vi "Main FPGA 5-axis with 5AxisLimitU8 48DIO.vi"() -> ()   [LabVIEW 2013]
uses:
  <vilib>/Motion/MotorControl/_s/nism.interpretControlRegister.stateTransition.ctl
  <vilib>/Platform/TimedLoop/XDataNode/timing_clust.ctl
  <vilib>/Platform/TimedLoop/XDataNode/nitl_modes.ctl
  <vilib>/Platform/TimedLoop/XDataNode/wakeup.ctl
  <vilib>/Motion/MotorControl/_s/nism.digitalInputs.portA.ctl
  <vilib>/rvi/Emulation/niFpgaSctlEmulationGetInTimedLoop.vi
  <vilib>/rvi/Emulation/niFpgaEmulationReportErrorSimple.vi
  <vilib>/rvi/Emulation/niFpgaGetClockAttributes.vi
  <vilib>/rvi/Emulation/niFpgaCriticalErrorInLSC.vi
  Global FPGA.vi
  <vilib>/rvi/eio/common/nirviEmuTemplateMethod_errors.vi
  <vilib>/Motion/SoftMotion/Synchronization/nism.rioScan.generateSyncScan.vi
  <vilib>/rvi/Emulation/niFpgaProcessEmulError.vi
  <vilib>/Motion/MotorControl/_s/nism.interpretControlRegister.indexed.vi
  <vilib>/Motion/MotorControl/_s/nism.generateStatusRegister.indexed.vi
  <vilib>/Motion/MotorControl/_s/nism.mdo.read.positionLoopSyncData.vi
  <vilib>/Motion/MotorControl/_s/nism.mdo.read.splineData.vi
  <vilib>/Motion/MotorControl/_s/nism.splineInterpolation.fxp.3.index.vi
  <vilib>/Motion/MotorControl/_s/nism.mdo.handler.indexed.vi
  <vilib>/Motion/MotorControl/_s/nism.interpretDIOControl.portA.single.2.vi
  <vilib>/Motion/MotorControl/_s/nism.generateDIOStatus.portA.single.vi
  <vilib>/Platform/TimedLoop/XDataNode/XDataNode.xnode
  <vilib>/eio/EIONode/EIONode.xnode
  <vilib>/Motion/MotorControl/NI_SoftMotion_MotorControlIP.lvlib
  <vilib>/Platform/TimedLoop/XDataNode/XDNodeRunTimeDep.lvlib
  <vilib>/Motion/SoftMotion/Synchronization/NI_SoftMotion_Synchronization.lvlib
panel:
  out "DI (24bits)":u32
  in  "DO (24bits)":u32
  in  "Axis Digital Input":u8[](array[numeric])=[0, 0, 0, 0, 0]
  out "Axis Positions":fxp<+/-,64,32>[](array[numeric])
  in  "STEP or CW? (T=STEP)":bool
  out "Drive Enable":bool[](array[boolean])
  in  "Enable Watchdog":bool
  in  "Pet Watchdog":bool
  in  "Watchdog Timeout Period (ticks)":u64=40000000 format="%.0p"
  out "Watchdog Timed Out?":bool
  out "Time Since Last Pet":u64
  in  "Enable value":bool
  in  "Drive Enable override?":bool
  out "State":T1=enum."Start --> Initializing" caption="state transition"
  in  "Sync Value":bool
  in  "Sync Enable override?":bool
  in  "Invert direction?":bool
  out "Sync is Fault":bool
  out "Sync is Locked":bool
  in  "minimum pulse":u16=40
  # "Synchronization Loop"
  # "Control Status Loop"
  # "Notes: \n1. This VI provides the communication interface between the NI SoftMotion Engine and the LabVIEW FPGA Module. You must compile this VI for a specific FPGA target before use. After compiling, run the VI before running any of the Express VI examples. For information on moving this example to another FPGA target, refer to ni.com/info and enter info code fpgaex.\n\n2. Only use the Reset Axis button if you are unable to communicate with the axis by any other means. This button resets the device state machine and other VIs to a known state. After resetting the axis, switch the NI Scan Engine from Active Mode to Configuration Mode, then back to Active Mode, before attempting to enable the axis."
  # "(These two buttons \nare for testing\npurposes.)"
  # "(These two buttons \nare for testing\npurposes.)"
  # "Step/Direction Loop"
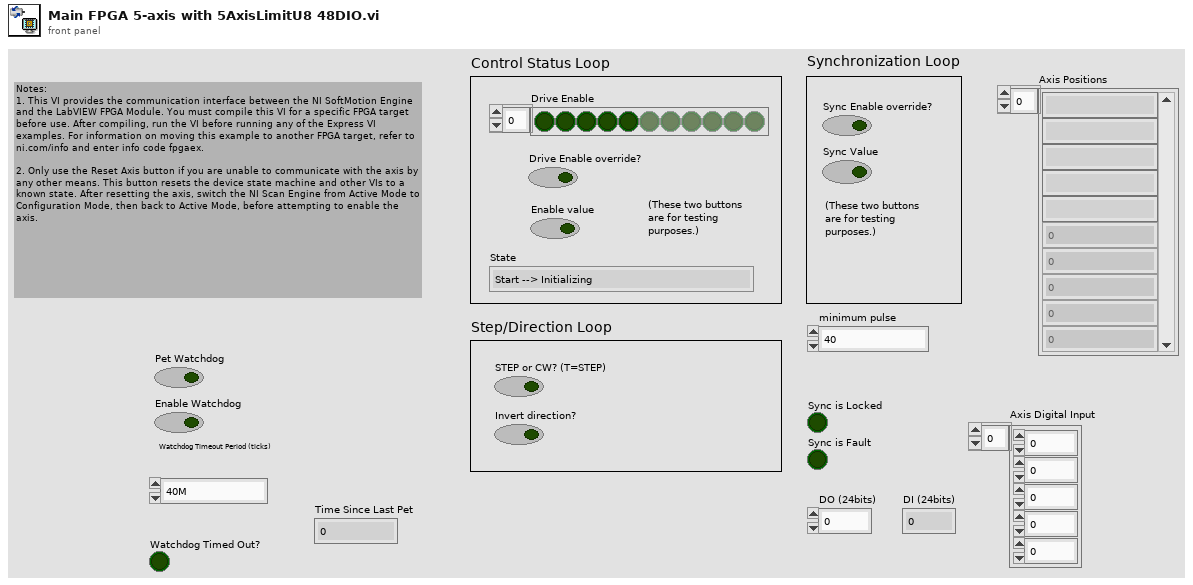
[diagram p1: front panel]
types:
  T1 = typedef "NI_SoftMotion_MotorControlIP.lvlib/nism.interpretControlRegister.stateTransition.ctl" = enum8{"Invalid", "Start --> Initializing", "Initializing --> Disabled", "Disabled --> Ready To Switch On", "Ready To Switch On --> Switched On", "Ready To Switch On --> Disable", "Switched On --> Operation Enable", "Switched On --> Ready To Switch On", "Switched On --> Disabled", "Operation Enable --> Switched On", "Operation Enable --> Ready To Switch On", "Operation Enable --> Disabled", "Fault --> Disabled", "Any --> Fault", "None"}
  T2 = typedef "NI_SoftMotion_MotorControlIP.lvlib/nism.mdo.splineData.ctl" = cluster{"spline type":T3, "traj per/spline per":u16, "spline per/traj per":fxp<+,32,0>}
  T3 = typedef "nism.splineInterpolation.type.ctl" = u16
  T4 = typedef "NI_SoftMotion_Synchronization.lvlib/nism.softmotionScan.timerConfig.ctl" = cluster{"Target Period (clocks)":u16, "Host Period / Target Period":u16}
  T5 = typedef "NI_SoftMotion_MotorControlIP.lvlib/nism.digitalInputs.portA.ctl" = cluster{"reverse limit":bool, "forward limit":bool, "home switch":bool, "digital input 0":bool, "digital input 1":bool, "digital input 2":bool, "digital input 3":bool}
  T6 = typedef "NI_SoftMotion_MotorControlIP.lvlib/nism.dio.portA.config.2.ctl" = cluster{"digital filter (us)":u16[], "safe state":enum16{"Low", "High", "No Change"}[]}
  T7 = typedef "XDNodeRunTimeDep.lvlib/timing_clust.ctl" = cluster{"Expected End [f-1]":u64, "Actual End [f-1]":u64, "Finished Late? [f-1]":bool, "Expected End [i-1]":u64, "Actual End [i-1]":u64, "Finished Late? [i-1]":bool, "Expected Start [i]":u64, "Actual Start [i]":u64, "Expected Start [f]":u64, "Actual Start [f]":u64, "Source Name":string, "Structure Name":string, "Period":i64, "Deadline":i64, "Offset":i64, "Start":i64, "Priority":i32, "Timeout":i32, "Mode":T8, "Wakeup Reason":T9, "Error":errorcluster, "Source Type":string, "Secondary Source Type":string, "Global End Time":u64, "Global Start Time":u64, "Frame Duration":u64, "Iteration Duration":u64, "Assigned CPU":i32, "I/O Scan Engine Mode":u32}
  T8 = typedef "XDNodeRunTimeDep.lvlib/nitl_modes.ctl" = enum32{"No Change", "Process missed periods, maintain original phase", "Discard missed periods, maintain original phase", "Process missed periods, ignore original phase", "Discard missed periods, ignore original phase"}
  T9 = typedef "XDNodeRunTimeDep.lvlib/wakeup.ctl" = enum32{"Normal", "Aborted", "Asynchronous wakeup", "Timing source error", "Timed loop error", "Timeout"}
  T10 = typedef "NI_SoftMotion_Synchronization.lvlib/nism.softmotionScan.timerControl.ctl" = cluster{"SM Scan":bool, "SM Scan Count":u32, "SM Scan Enabled":bool}
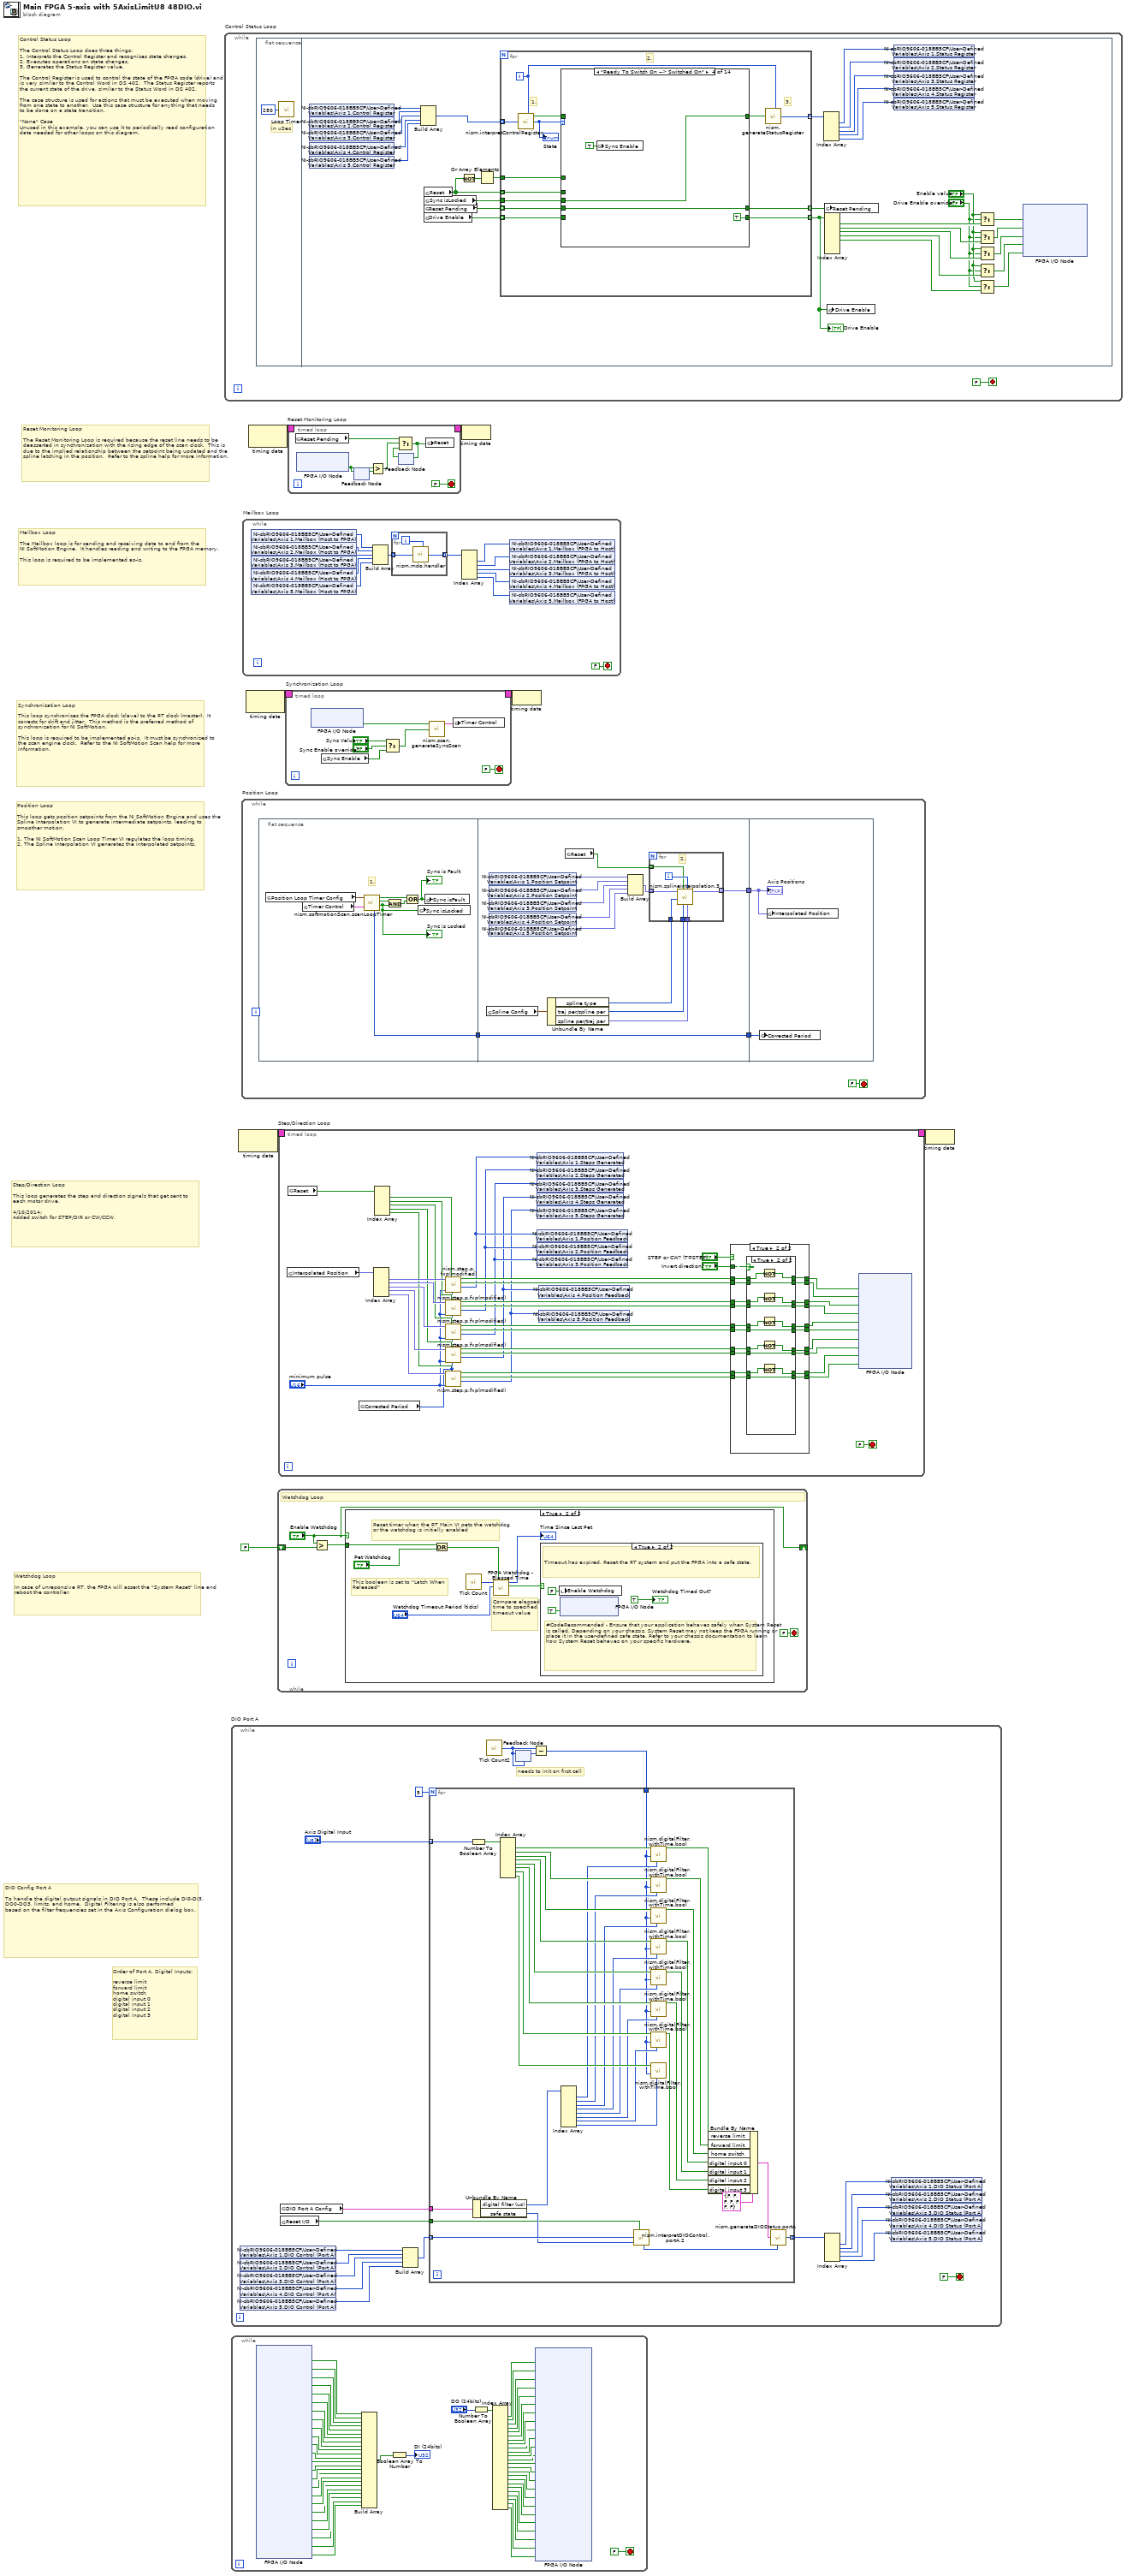
[diagram p0: block diagram]
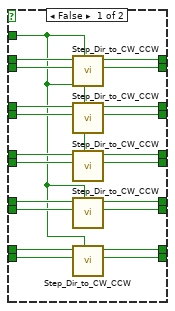
[diagram p4: hidden frame]
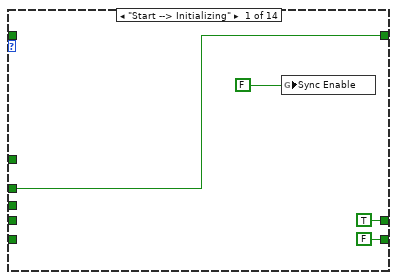
[diagram p6: hidden frame]
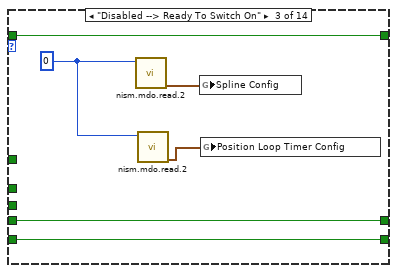
[diagram p8: hidden frame]
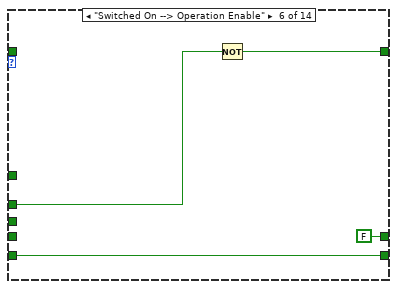
[diagram p10: hidden frame]
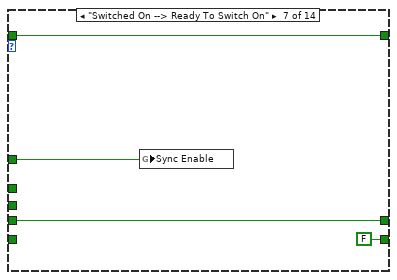
[diagram p11: hidden frame]
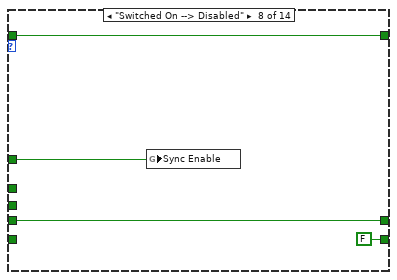
[diagram p12: hidden frame]
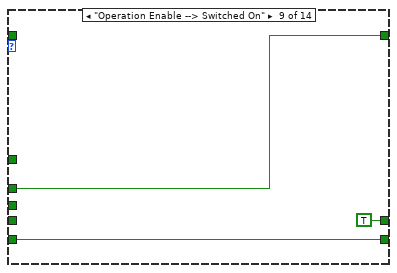
[diagram p13: hidden frame]
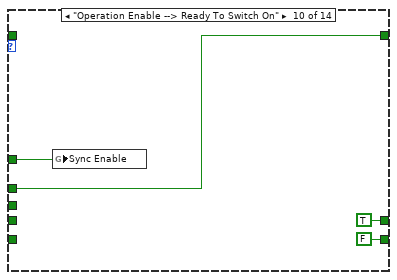
[diagram p14: hidden frame]
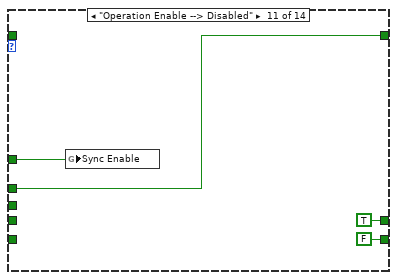
[diagram p15: hidden frame]
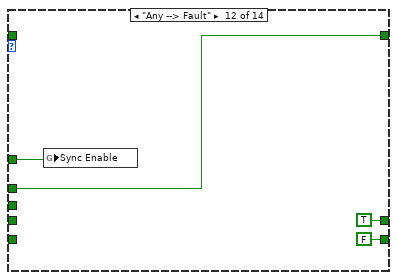
[diagram p16: hidden frame]
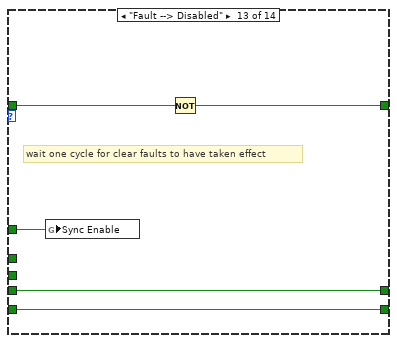
[diagram p17: hidden frame]
diagram:
  # "DIO Config Port A\n\nTo handle the digital output signals in DIO Port A.  These include DI0-DI3, DO0-DO3, limits, and home.  Digital Filtering is also performed\nbased on the filter frequencies set in the Axis Configuration dialog box."
  # "Order of Port A, Digital Inputs:\n\nreverse limit\nforward limit\nhome switch\ndigital input 0\ndigital input 1\ndigital input 2\ndigital input 3"
  # "Watchdog Loop\n\nIn case of unreponsive RT, the FPGA will assert the \"System Reset\" line and reboot the controller."
  # "Step/Direction Loop\n\nThis loop generates the step and direction signals that get sent to \neach motor drive.\n\n4/10/2014:\nAdded switch for STEP/DIR or CW/CCW."
  # "Position Loop\n\nThis loop gets position setpoints from the NI SoftMotion Engine and uses the Spline Interpolation VI to generate intermediate setpoints, leading to smoother motion.\n\n1. The NI SoftMotion Scan Loop Timer VI regulates the loop timing. \n2. The Spline Interpolation VI generates the interpolated setpoints."
  # "Synchronization Loop\n\nThis loop synchronizes the FPGA clock (slave) to the RT clock (master).  It corrects for drift and jitter.  This method is the preferred method of synchronization for NI SoftMotion.\n\nThis loop is required to be implemented as-is.  It must be synchronized to the scan engine clock.  Refer to the NI SoftMotion Scan help for more information."
  # "Mailbox Loop\n\nThe Mailbox loop is for sending and receiving data to and from the \nNI SoftMotion Engine.  It handles reading and writing to the FPGA memory.\n\nThis loop is required to be implemented as-is."
  # "Reset Monitoring Loop\n\nThe Reset Monitoring Loop is required because the reset line needs to be deasserted in synchronization with the rising edge of the scan clock.  This is due to the implied relationship between the setpoint being updated and the spline latching in the position.  Refer to the spline help for more information."
  # "Control Status Loop\n\nThe Control Status Loop does three things:\n1. Interprets the Control Register and recognizes state changes.\n2. Executes operations on state changes.\n3. Generates the Status Register value.\n\nThe Control Register is used to control the state of the FPGA code (drive) and is very similar to the Control Word in DS 402.  The Status Register reports the current state of the drive, similar to the Status Word in DS 402.\n\nThe case structure is used for actions that must be executed when moving from one state to another.  Use this case structure for anything that needs to be done on a state transition.\n\n\"None\" Case\nUnused in this example, you can use it to periodically read configuration data needed for other loops on this diagram."
  n1 = while "Control Status Loop" {
    stop <- FALSE stop-if-true
    n2 = flat-sequence {
      frame #0 {
        # "in uSec"
        n3 = call "Loop Timer"("Count(uSec)"=u32 250) -> ()  [unwired: 1 out]
      }
      frame #1 {
        n4 = shared-variable "NI-sbRIO9606-018BB5CF\\User-Defined Variables\\Axis 1.Control Register"() -> (w31:u32)  [unwired: 1 in, 1 out]
        n5 = shared-variable "NI-sbRIO9606-018BB5CF\\User-Defined Variables\\Axis 2.Control Register"() -> (w30:u32)  [unwired: 1 in, 1 out]
        n6 = shared-variable "NI-sbRIO9606-018BB5CF\\User-Defined Variables\\Axis 3.Control Register"() -> (w29:u32)  [unwired: 1 in, 1 out]
        n7 = shared-variable "NI-sbRIO9606-018BB5CF\\User-Defined Variables\\Axis 4.Control Register"() -> (w28:u32)  [unwired: 1 in, 1 out]
        n8 = shared-variable "NI-sbRIO9606-018BB5CF\\User-Defined Variables\\Axis 5.Control Register"() -> (w27:u32)  [unwired: 1 in, 1 out]
        n9 = Build Array(w31, w30, w29, w28, w27) -> (w40:u32[])
        n10 = global read "Global FPGA.vi" "Reset Pending"() -> (w35:bool[])
        n11 = global read "Global FPGA.vi" "Drive Enable"() -> (w34:bool[])
        n12 = global read "Global FPGA.vi" "Reset"() -> (w36:bool[])
        n13 = global read "Global FPGA.vi" "Sync isLocked"() -> (w41:bool)
        n14 = Not(x=w36) -> (.not. x?=w38:bool[])
        n15 = Or Array Elements(Boolean array=w38) -> (logical OR=w37:bool)
        n16 = for {
          tunnel: w36 -> [w49] mode=indexing
          tunnel: w41 -> [w48]
          tunnel: w40 -> [w50] mode=indexing
          tunnel: [w47] -> w32 mode=indexing
          tunnel: [w46] -> w39 mode=indexing
          tunnel: [w45] -> w33 mode=indexing
          tunnel: w37 -> [w44]
          tunnel: w35 -> [w43] mode=indexing
          tunnel: w34 -> [w42] mode=indexing
          i -> [w51]
          # "3."
          # "2."
          # "1."
          n17 = call-poly <vilib>:"nism.interpretControlRegister.vi"("control register"=w50, "axis index"=w51) -> ("transition occurred"=w52:bool, "state transition"=w53:T1)  [unwired: 6 in]
          "State" <- w53
          n18 = case shown="\"Ready To Switch On --> Switched On\"" w53 {
            tunnel: w52 -> [_ w61 w67 _ w74 _ w82 w86 _ _ _ _ w106 _]
            tunnel: [w58 w61 w67 w69 w74 w78 w82 w86 w88 w91 w95 w99 w105 _] -> w54
            tunnel: w49 -> [w58 _ _ _ _ w77 _ _ w88 w91 w95 w99 _ _]
            tunnel: w48 -> [_ _ _ w69 _ _ _ _ _ _ _ _ _ _]
            tunnel: [TRUE ("Write.Reset Pending") w60 w63 w68 w73 FALSE ("Write.Reset Pending") w79 w83 TRUE ("Write.Reset Pending") TRUE ("Write.Reset Pending") TRUE ("Write.Reset Pending") TRUE ("Write.Reset Pending") w103 w108] -> w46
            tunnel: [FALSE ("Write.Drive Enable") w59 w62 TRUE ("Write.Drive Enable") w72 w75 FALSE ("Write.Drive Enable") FALSE ("Write.Drive Enable") w87 FALSE ("Write.Drive Enable") FALSE ("Write.Drive Enable") FALSE ("Write.Drive Enable") w102 w107] -> w45
            tunnel: w44 -> [_ _ _ _ _ _ w80 w84 _ w90 w94 w98 w104 _]
            tunnel: w43 -> [_ w60 w63 w68 w73 _ w79 w83 _ _ _ _ w103 w108]
            tunnel: w42 -> [_ w59 w62 _ w72 w75 _ _ w87 _ _ _ w102 w107]
            frame "Start --> Initializing" {
              n19 = global write "Global FPGA.vi" "Sync Enable"(FALSE ("Sync Enable")) -> ()
            }
            frame "Initializing --> Disabled" {
            }
            frame "Disabled --> Ready To Switch On" {
              w65 = 0 ("axis index")
              n20 = call-poly <vilib>:"nism.mdo.read.2.vi"("axis index"=w65) -> ("spline"=w66:T2)  [unwired: 10 in]
              n21 = call-poly <vilib>:"nism.mdo.read.2.vi"("axis index"=w65) -> ("position loop sync"=w64:T4)  [unwired: 10 in]
              n22 = global write "Global FPGA.vi" "Spline Config"(w66) -> ()
              n23 = global write "Global FPGA.vi" "Position Loop Timer Config"(w64) -> ()
            }
            frame "Ready To Switch On --> Switched On" {
              n24 = global write "Global FPGA.vi" "Sync Enable"(TRUE ("Sync Enable")) -> ()
            }
            frame "Ready To Switch On --> Disable" {
            }
            frame "Switched On --> Operation Enable" {
              n25 = Not(x=w77) -> (.not. x?=w78:bool)
            }
            frame "Switched On --> Ready To Switch On" {
              n26 = global write "Global FPGA.vi" "Sync Enable"(w80) -> ()
            }
            frame "Switched On --> Disabled" {
              n27 = global write "Global FPGA.vi" "Sync Enable"(w84) -> ()
            }
            frame "Operation Enable --> Switched On" {
            }
            frame "Operation Enable --> Ready To Switch On" {
              n28 = global write "Global FPGA.vi" "Sync Enable"(w90) -> ()
            }
            frame "Operation Enable --> Disabled" {
              n29 = global write "Global FPGA.vi" "Sync Enable"(w94) -> ()
            }
            frame "Any --> Fault" {
              n30 = global write "Global FPGA.vi" "Sync Enable"(w98) -> ()
            }
            frame "Fault --> Disabled" {
              # "wait one cycle for clear faults to have taken effect"
              n31 = global write "Global FPGA.vi" "Sync Enable"(w104) -> ()
              n32 = Not(x=w106) -> (.not. x?=w105:bool)
            }
            frame "None", Default {
            }
          }
          n33 = call-poly <vilib>:"nism.generateStatusRegister.vi"("transition success"=w54, "axis index"=w51) -> ("status register"=w47:u32)  [unwired: 7 in]
        }
        "Drive Enable" <- w33
        n34 = Index Array(array=w32) -> (element #1=w26:u32, element #2=w25:u32, element #3=w24:u32, element #4=w23:u32, element #5=w22:u32)  [unwired: 5 in]
        n35 = global write "Global FPGA.vi" "Reset Pending"(w39) -> ()
        n36 = Index Array(array=w33) -> (element #1=w21:bool, element #2=w19:bool, element #3=w17:bool, element #4=w15:bool, element #5=w13:bool)  [unwired: 8 in, 3 out]
        n37 = global write "Global FPGA.vi" "Drive Enable"(w33) -> ()
        n38 = shared-variable "NI-sbRIO9606-018BB5CF\\User-Defined Variables\\Axis 1.Status Register"(w26) -> ()  [unwired: 1 in, 1 out]
        n39 = shared-variable "NI-sbRIO9606-018BB5CF\\User-Defined Variables\\Axis 2.Status Register"(w25) -> ()  [unwired: 1 in, 1 out]
        n40 = shared-variable "NI-sbRIO9606-018BB5CF\\User-Defined Variables\\Axis 3.Status Register"(w24) -> ()  [unwired: 1 in, 1 out]
        n41 = shared-variable "NI-sbRIO9606-018BB5CF\\User-Defined Variables\\Axis 4.Status Register"(w23) -> ()  [unwired: 1 in, 1 out]
        n42 = shared-variable "NI-sbRIO9606-018BB5CF\\User-Defined Variables\\Axis 5.Status Register"(w22) -> ()  [unwired: 1 in, 1 out]
        n43 = Select(t="Enable value", s="Drive Enable override?", f=w21) -> (s? t:f=w20:bool)
        n44 = Select(t="Enable value", s="Drive Enable override?", f=w19) -> (s? t:f=w18:bool)
        n45 = Select(t="Enable value", s="Drive Enable override?", f=w17) -> (s? t:f=w16:bool)
        n46 = Select(t="Enable value", s="Drive Enable override?", f=w15) -> (s? t:f=w14:bool)
        n47 = Select(t="Enable value", s="Drive Enable override?", f=w13) -> (s? t:f=w12:bool)
        n48 = xnode "FPGA I/O Node"("Axis1_Servo On"=w20, "Axis2_Servo On"=w18, "Axis3_Servo On"=w16, "Axis4_Servo On"=w14, "Axis5_Servo On"=w12) -> ()  [unwired: 5 in, 5 out]
      }
    }
  }
  n49 = while "DIO Port A" {
    stop <- FALSE stop-if-true
    # "needs to init on first call"
    n50 = shared-variable "NI-sbRIO9606-018BB5CF\\User-Defined Variables\\Axis 1.DIO Control (Port A)"() -> (w125:u32)  [unwired: 1 in, 1 out]
    n51 = shared-variable "NI-sbRIO9606-018BB5CF\\User-Defined Variables\\Axis 2.DIO Control (Port A)"() -> (w124:u32)  [unwired: 1 in, 1 out]
    n52 = shared-variable "NI-sbRIO9606-018BB5CF\\User-Defined Variables\\Axis 3.DIO Control (Port A)"() -> (w123:u32)  [unwired: 1 in, 1 out]
    n53 = shared-variable "NI-sbRIO9606-018BB5CF\\User-Defined Variables\\Axis 4.DIO Control (Port A)"() -> (w122:u32)  [unwired: 1 in, 1 out]
    n54 = shared-variable "NI-sbRIO9606-018BB5CF\\User-Defined Variables\\Axis 5.DIO Control (Port A)"() -> (w121:u32)  [unwired: 1 in, 1 out]
    n55 = global read "Global FPGA.vi" "DIO Port A Config"() -> (w109:T6)
    n56 = global read "Global FPGA.vi" "Reset I/O"() -> (w110:bool)
    n57 = Build Array(w125, w124, w123, w122, w121) -> (w120:u32[])
    n58 = call "Tick Count2"() -> ("Tick Count(uSec)"=w113:u16)
    n59 = feedback #1(w113) -> (w112:u16)
    n60 = feedback-in #1(w113) -> ()
    n61 = Subtract(x=w113, y=w112) -> (x-y=w111:u16)
    n62 = for {
      N: 5 -> [_]
      tunnel: [w162] -> w114 mode=indexing
      tunnel: w120 -> [w161] mode=indexing
      tunnel: w109 -> [w158]
      tunnel: w110 -> [w156]
      tunnel: "Axis Digital Input" -> [w130] mode=indexing
      tunnel: w111 -> [w129]
      n63 = Number To Boolean Array(number=w130) -> (Boolean array=w155:bool[])
      n64 = Unbundle By Name(w158) -> ("digital filter (us)"=w138:u16[], "safe state"=w157:enum16{"Low", "High", "No Change"}[])
      n65 = Index Array(array=w155) -> (element #1=w154:bool, element #2=w147:bool, element #3=w148:bool, element #4=w149:bool, element #5=w150:bool, element #6=w151:bool, element #7=w152:bool, element #8=w153:bool)  [unwired: 8 in]
      n66 = Index Array(array=w138) -> (element #1=w139:u16, element #2=w140:u16, element #3=w141:u16, element #4=w142:u16, element #5=w143:u16, element #6=w144:u16, element #7=w145:u16, element #8=w146:u16)  [unwired: 8 in]
      n67 = call-poly <vilib>:"nism.interpretDIOControl.portA.2.vi"("reset"=w156, "dio control(port a)"=w161, "safe state"=w157) -> ("reset latches"=w163:u8)  [unwired: 5 in, 1 out]
      n68 = call <vilib>:"nism.digitalFilter.withTime.bool.vi"("filter value"=w139, "delta time"=w129, "input signal"=w154) -> ("output signal"=w137:bool)  [unwired: 8 in]
      n69 = call <vilib>:"nism.digitalFilter.withTime.bool.vi"("filter value"=w140, "delta time"=w129, "input signal"=w147) -> ("output signal"=w136:bool)  [unwired: 8 in]
      n70 = call <vilib>:"nism.digitalFilter.withTime.bool.vi"("filter value"=w141, "delta time"=w129, "input signal"=w148) -> ("output signal"=w135:bool)  [unwired: 8 in]
      n71 = call <vilib>:"nism.digitalFilter.withTime.bool.vi"("filter value"=w142, "delta time"=w129, "input signal"=w149) -> ("output signal"=w134:bool)  [unwired: 8 in]
      n72 = call <vilib>:"nism.digitalFilter.withTime.bool.vi"("filter value"=w143, "delta time"=w129, "input signal"=w150) -> ("output signal"=w133:bool)  [unwired: 8 in]
      n73 = call <vilib>:"nism.digitalFilter.withTime.bool.vi"("filter value"=w144, "delta time"=w129, "input signal"=w151) -> ("output signal"=w132:bool)  [unwired: 8 in]
      n74 = call <vilib>:"nism.digitalFilter.withTime.bool.vi"("filter value"=w145, "delta time"=w129, "input signal"=w152) -> ("output signal"=w131:bool)  [unwired: 8 in]
      n75 = call <vilib>:"nism.digitalFilter.withTime.bool.vi"("filter value"=w146, "delta time"=w129, "input signal"=w153) -> ()  [unwired: 8 in, 1 out]
      n76 = Bundle By Name(cluster=T5 {"reverse limit"=FALSE, "forward limit"=FALSE, "home switch"=FALSE, "digital input 0"=FALSE, "digital input 1"=FALSE, "digital input 2"=FALSE, "digital input 3"=FALSE} ("$(driveInterface.digitalInputs.shortName)"), "reverse limit"=w137, "forward limit"=w136, "home switch"=w135, "digital input 0"=w134, "digital input 1"=w133, "digital input 2"=w132, "digital input 3"=w131) -> (w159:T5)
      n77 = call-poly <vilib>:"nism.generateDIOStatus.portA.vi"("digital inputs"=w159, "reset latches"=w163) -> ("dio status(port a)"=w162:u32)  [unwired: 7 in]
    }
    n78 = Index Array(array=w114) -> (element #1=w119:u32, element #2=w118:u32, element #3=w117:u32, element #4=w116:u32, element #5=w115:u32)  [unwired: 5 in]
    n79 = shared-variable "NI-sbRIO9606-018BB5CF\\User-Defined Variables\\Axis 1.DIO Status (Port A)"(w119) -> ()  [unwired: 1 in, 1 out]
    n80 = shared-variable "NI-sbRIO9606-018BB5CF\\User-Defined Variables\\Axis 2.DIO Status (Port A)"(w118) -> ()  [unwired: 1 in, 1 out]
    n81 = shared-variable "NI-sbRIO9606-018BB5CF\\User-Defined Variables\\Axis 3.DIO Status (Port A)"(w117) -> ()  [unwired: 1 in, 1 out]
    n82 = shared-variable "NI-sbRIO9606-018BB5CF\\User-Defined Variables\\Axis 4.DIO Status (Port A)"(w116) -> ()  [unwired: 1 in, 1 out]
    n83 = shared-variable "NI-sbRIO9606-018BB5CF\\User-Defined Variables\\Axis 5.DIO Status (Port A)"(w115) -> ()  [unwired: 1 in, 1 out]
  }
  n84 = while {
    stop <- FALSE stop-if-true
    n85 = xnode "FPGA I/O Node"() -> ("RMC/DIO20"=w216:bool, "RMC/DIO21"=w215:bool, "RMC/DIO22"=w214:bool, "RMC/DIO23"=w213:bool, "RMC/DIO24"=w212:bool, "RMC/DIO25"=w211:bool, "RMC/DIO26"=w210:bool, "RMC/DIO27"=w209:bool, "RMC/DIO28"=w208:bool, "RMC/DIO29"=w207:bool, "RMC/DIO30"=w206:bool, "RMC/DIO31"=w205:bool, "RMC/DIO33"=w204:bool, "RMC/DIO34"=w203:bool, "RMC/DIO35"=w202:bool, "RMC/DIO36"=w201:bool, "RMC/DIO37"=w200:bool, "RMC/DIO38"=w199:bool, "RMC/DIO39"=w198:bool, "RMC/DIO40"=w197:bool, "RMC/DIO41"=w196:bool, "RMC/DIO42"=w195:bool, "RMC/DIO43"=w194:bool, "RMC/DIO44"=w193:bool)  [unwired: 24 in, 24 out]
    n86 = Build Array(w216, w215, w214, w213, w212, w211, w210, w209, w208, w207, w206, w205, w204, w203, w202, w201, w200, w199, w198, w197, w196, w195, w194, w193) -> (w166:bool[])
    n87 = Boolean Array To Number(Boolean array=w166) -> (number=→"DI (24bits)":u32)
    n88 = Number To Boolean Array(number="DO (24bits)") -> (Boolean array=w191:bool[])
    n89 = Index Array(array=w191) -> (element #1=w192:bool, element #2=w190:bool, element #3=w189:bool, element #4=w188:bool, element #5=w187:bool, element #6=w186:bool, element #7=w185:bool, element #8=w184:bool, element #9=w183:bool, element #10=w182:bool, element #11=w181:bool, element #12=w180:bool, element #13=w179:bool, element #14=w178:bool, element #15=w177:bool, element #16=w176:bool, element #17=w175:bool, element #18=w174:bool, element #19=w173:bool, element #20=w172:bool, element #21=w171:bool, element #22=w170:bool, element #23=w169:bool, element #24=w168:bool)  [unwired: 24 in]
    n90 = xnode "FPGA I/O Node"("RMC/DIO45"=w192, "RMC/DIO46"=w190, "RMC/DIO47"=w189, "RMC/DIO49"=w188, "RMC/DIO50"=w187, "RMC/DIO51"=w186, "RMC/DIO52"=w185, "RMC/DIO53"=w184, "RMC/DIO54"=w183, "RMC/DIO55"=w182, "RMC/DIO56"=w181, "RMC/DIO57"=w180, "RMC/DIO58"=w179, "RMC/DIO59"=w178, "RMC/DIO60"=w177, "RMC/DIO61"=w176, "RMC/DIO62"=w175, "RMC/DIO63"=w174, "RMC/DIO70"=w173, "RMC/DIO77"=w172, "RMC/DIO82"=w171, "RMC/DIO83"=w170, "RMC/DIO84"=w169, "RMC/DIO89"=w168) -> ()  [unwired: 24 in, 24 out]
  }
  n91 = node-c288() -> (w7:T7)  [unwired: 1 in]
  n92 = while "Position Loop" {
    stop <- FALSE stop-if-true
    n93 = flat-sequence {
      tunnel: [w221] -> w217
      tunnel: [w235] -> w219
      tunnel: [w234] -> w218
      tunnel: w217 -> [w234]
      tunnel: w219 -> [w249]
      tunnel: w218 -> [w250]
      frame #0 {
        # "1."
        n94 = global read "Global FPGA.vi" "Position Loop Timer Config"() -> (w223:T4)
        n95 = global read "Global FPGA.vi" "Timer Control"() -> (w222:T10)
        n96 = call <vilib>:"nism.softmotionScan.scanLoopTimer.vi"("Timer Control"=w222, "Timer Config"=w223) -> ("Scan Running?"=w225:bool, "Finished Late?"=w227:bool, "Fault Occurred?"=w228:bool, "Corrected Period"=w221:u16)  [unwired: 5 in, 1 out]
        "Sync is Locked" <- w225
        n97 = Compound Arithmetic op=AND(w227, w225) -> (w226:bool)
        n98 = Compound Arithmetic op=OR(w228, w226) -> (w224:bool)
        "Sync is Fault" <- w224
        n99 = global write "Global FPGA.vi" "Sync isLocked"(w225) -> ()
        n100 = global write "Global FPGA.vi" "Sync isFault"(w224) -> ()
      }
      frame #1 {
        n101 = global read "Global FPGA.vi" "Spline Config"() -> (w237:T2)
        n102 = shared-variable "NI-sbRIO9606-018BB5CF\\User-Defined Variables\\Axis 1.Position Setpoint"() -> (w233:fxp<+/-,64,32>)  [unwired: 1 in, 1 out]
        n103 = shared-variable "NI-sbRIO9606-018BB5CF\\User-Defined Variables\\Axis 2.Position Setpoint"() -> (w232:fxp<+/-,64,32>)  [unwired: 1 in, 1 out]
        n104 = shared-variable "NI-sbRIO9606-018BB5CF\\User-Defined Variables\\Axis 3.Position Setpoint"() -> (w231:fxp<+/-,64,32>)  [unwired: 1 in, 1 out]
        n105 = shared-variable "NI-sbRIO9606-018BB5CF\\User-Defined Variables\\Axis 4.Position Setpoint"() -> (w230:fxp<+/-,64,32>)  [unwired: 1 in, 1 out]
        n106 = shared-variable "NI-sbRIO9606-018BB5CF\\User-Defined Variables\\Axis 5.Position Setpoint"() -> (w229:fxp<+/-,64,32>)  [unwired: 1 in, 1 out]
        n107 = Unbundle By Name(w237) -> ("spline type"=w241:T3, "traj per/spline per"=w240:u16, "spline per/traj per"=w239:fxp<+,32,0>)
        n108 = global read "Global FPGA.vi" "Reset"() -> (w236:bool[])
        n109 = Build Array(w233, w232, w231, w230, w229) -> (w238:fxp<+/-,64,32>[])
        n110 = for {
          tunnel: w241 -> [w248]
          tunnel: w240 -> [w247]
          tunnel: w239 -> [w246]
          tunnel: w236 -> [w243] mode=indexing
          tunnel: w238 -> [w245] mode=indexing
          tunnel: [w242] -> w235 mode=indexing
          i -> [w244]
          # "2."
          n111 = call-poly <vilib>:"nism.splineInterpolation.3.vi"("1 / calls per sample"=w246, "index"=w244, "calls per sample"=w247, "reset"=w243, "spline type"=w248, "x"=w245) -> ("xi"=w242:fxp<+/-,64,32>)  [unwired: 5 in]
        }
      }
      frame #2 {
        n112 = global write "Global FPGA.vi" "Corrected Period"(w250) -> ()
        n113 = global write "Global FPGA.vi" "Interpolated Position"(w249) -> ()
        "Axis Positions" <- w249
      }
    }
  }
  n114 = while "Mailbox Loop" {
    stop <- FALSE stop-if-true
    n115 = shared-variable "NI-sbRIO9606-018BB5CF\\User-Defined Variables\\Axis 1.Mailbox (Host to FPGA)"() -> (w260:u64)  [unwired: 1 in, 1 out]
    n116 = shared-variable "NI-sbRIO9606-018BB5CF\\User-Defined Variables\\Axis 2.Mailbox (Host to FPGA)"() -> (w259:u64)  [unwired: 1 in, 1 out]
    n117 = shared-variable "NI-sbRIO9606-018BB5CF\\User-Defined Variables\\Axis 3.Mailbox (Host to FPGA)"() -> (w258:u64)  [unwired: 1 in, 1 out]
    n118 = shared-variable "NI-sbRIO9606-018BB5CF\\User-Defined Variables\\Axis 4.Mailbox (Host to FPGA)"() -> (w257:u64)  [unwired: 1 in, 1 out]
    n119 = shared-variable "NI-sbRIO9606-018BB5CF\\User-Defined Variables\\Axis 5.Mailbox (Host to FPGA)"() -> (w256:u64)  [unwired: 1 in, 1 out]
    n120 = Build Array(w260, w259, w258, w257, w256) -> (w262:u64[])
    n121 = for {
      tunnel: w262 -> [w266] mode=indexing
      tunnel: [w265] -> w261 mode=indexing
      i -> [w264]
      n122 = call-poly <vilib>:"nism.mdo.handler.vi"("mbox (host to fpga)"=w266, "axis index"=w264) -> ("mbox (fpga to host)"=w265:u64)  [unwired: 7 in]
    }
    n123 = Index Array(array=w261) -> (element #1=w255:u64, element #2=w254:u64, element #3=w253:u64, element #4=w252:u64, element #5=w251:u64)  [unwired: 5 in]
    n124 = shared-variable "NI-sbRIO9606-018BB5CF\\User-Defined Variables\\Axis 5.Mailbox (FPGA to Host)"(w251) -> ()  [unwired: 1 in, 1 out]
    n125 = shared-variable "NI-sbRIO9606-018BB5CF\\User-Defined Variables\\Axis 1.Mailbox (FPGA to Host)"(w255) -> ()  [unwired: 1 in, 1 out]
    n126 = shared-variable "NI-sbRIO9606-018BB5CF\\User-Defined Variables\\Axis 2.Mailbox (FPGA to Host)"(w254) -> ()  [unwired: 1 in, 1 out]
    n127 = shared-variable "NI-sbRIO9606-018BB5CF\\User-Defined Variables\\Axis 3.Mailbox (FPGA to Host)"(w253) -> ()  [unwired: 1 in, 1 out]
    n128 = shared-variable "NI-sbRIO9606-018BB5CF\\User-Defined Variables\\Axis 4.Mailbox (FPGA to Host)"(w252) -> ()  [unwired: 1 in, 1 out]
  }
  n129 = node-c288() -> (w5:T7)  [unwired: 1 in]
  n130 = node-c288() -> (w3:T7)  [unwired: 1 in]
  n131 = while "RT Watchdog Loop" {
    shift-right: ["Enable Watchdog"] -> _
    shift-left: FALSE ("Enable RT Watchdog") -> [w270]
    stop <- FALSE stop-if-true
    # "Watchdog Loop"
    n132 = Greater?(x="Enable Watchdog", y=w270) -> (0:w267:bool)
    n133 = case shown="True" "Enable Watchdog" {
      tunnel: w267 -> [_ w273]
      frame False {
        # "This loop has to be explicitly enabled from the RT Main VI.  This reduces the possiblity of an endless reboot cycle."
      }
      frame True {
        # "This boolean is set to \"Latch When Released\""
        # "Compare elapsed time to specified timeout value"
        # "Reset timer when the RT Main VI pets the watchdog or the watchdog is initially enabled"
        n134 = Or(x=w273, y="Pet Watchdog") -> (x .or. y?=w272:bool)
        n135 = call "Tick Count"() -> ("Tick Count(Ticks)"=w276:u32)
        n136 = call "FPGA Watchdog - Elapsed Time.vi"("Reset"=w272, "Timeout Period"="Watchdog Timeout Period (ticks)", "Current Time"=w276) -> ("Timeout"=w271:bool, "Elapsed Time"=→"Time Since Last Pet":u64)  [unwired: 7 in]
        n137 = case shown="True" w271 {
          frame False {
            # "Timeout has not expired."
          }
          frame True {
            # "#CodeRecommended - Ensure that your application behaves safely when System Reset is called. Depending on your chassis, System Reset may not keep the FPGA running or place it in the user-defined safe state. Refer to your chassis documentation to learn how System Reset behaves on your specific hardware."
            # "Timeout has expired. Reset the RT system and put the FPGA into a safe state."
            n138 = local write "Enable Watchdog"(FALSE ("Enable RT Watchdog")) -> ()
            n139 = xnode "FPGA I/O Node"("System Reset"=TRUE ("RT Reset on Watchdog Failure?")) -> ()  [unwired: 1 in, 1 out]
            "Watchdog Timed Out?" <- TRUE ("Watchdog Timed Out?")
          }
        }
      }
    }
  }
  n140 = timed-loop "Step/Direction Loop" {
    timing: w7 -> [_]
    timing-out: [_] -> w6
    stop <- FALSE stop-if-true
    n141 = global read "Global FPGA.vi" "Interpolated Position"() -> (w321:fxp<+/-,64,32>[])
    n142 = global read "Global FPGA.vi" "Reset"() -> (w315:bool[])
    n143 = global read "Global FPGA.vi" "Corrected Period"() -> (w281:u16)
    n144 = Index Array(array=w321) -> (element #1=w320:fxp<+/-,64,32>, element #2=w319:fxp<+/-,64,32>, element #3=w318:fxp<+/-,64,32>, element #4=w317:fxp<+/-,64,32>, element #5=w316:fxp<+/-,64,32>)  [unwired: 5 in]
    n145 = Index Array(array=w315) -> (element #1=w314:bool, element #2=w313:bool, element #3=w312:bool, element #4=w311:bool, element #5=w310:bool)  [unwired: 5 in]
    n146 = call "nism.step.p.fxp(modified).vi"("calls per sample"=w281, "reset"=w314, "minimum pulse"="minimum pulse", "position setpoint"=w320) -> ("steps generated"=w286:i32, "step"=w308:bool, "direction"=w309:bool)  [unwired: 4 in, 1 out]
    n147 = call "nism.step.p.fxp(modified).vi"("calls per sample"=w281, "reset"=w313, "minimum pulse"="minimum pulse", "position setpoint"=w319) -> ("steps generated"=w285:i32, "step"=w306:bool, "direction"=w307:bool)  [unwired: 4 in, 1 out]
    n148 = call "nism.step.p.fxp(modified).vi"("calls per sample"=w281, "reset"=w312, "minimum pulse"="minimum pulse", "position setpoint"=w318) -> ("steps generated"=w284:i32, "step"=w304:bool, "direction"=w305:bool)  [unwired: 4 in, 1 out]
    n149 = call "nism.step.p.fxp(modified).vi"("calls per sample"=w281, "reset"=w311, "minimum pulse"="minimum pulse", "position setpoint"=w317) -> ("steps generated"=w283:i32, "step"=w302:bool, "direction"=w303:bool)  [unwired: 4 in, 1 out]
    n150 = call "nism.step.p.fxp(modified).vi"("calls per sample"=w281, "reset"=w310, "minimum pulse"="minimum pulse", "position setpoint"=w316) -> ("steps generated"=w282:i32, "step"=w300:bool, "direction"=w301:bool)  [unwired: 4 in, 1 out]
    n151 = shared-variable "NI-sbRIO9606-018BB5CF\\User-Defined Variables\\Axis 1.Steps Generated"(w286) -> ()  [unwired: 1 in, 1 out]
    n152 = shared-variable "NI-sbRIO9606-018BB5CF\\User-Defined Variables\\Axis 2.Steps Generated"(w285) -> ()  [unwired: 1 in, 1 out]
    n153 = shared-variable "NI-sbRIO9606-018BB5CF\\User-Defined Variables\\Axis 3.Steps Generated"(w284) -> ()  [unwired: 1 in, 1 out]
    n154 = shared-variable "NI-sbRIO9606-018BB5CF\\User-Defined Variables\\Axis 4.Steps Generated"(w283) -> ()  [unwired: 1 in, 1 out]
    n155 = shared-variable "NI-sbRIO9606-018BB5CF\\User-Defined Variables\\Axis 5.Steps Generated"(w282) -> ()  [unwired: 1 in, 1 out]
    n156 = shared-variable "NI-sbRIO9606-018BB5CF\\User-Defined Variables\\Axis 1.Position Feedback"(w286) -> ()  [unwired: 1 in, 1 out]
    n157 = shared-variable "NI-sbRIO9606-018BB5CF\\User-Defined Variables\\Axis 2.Position Feedback"(w285) -> ()  [unwired: 1 in, 1 out]
    n158 = shared-variable "NI-sbRIO9606-018BB5CF\\User-Defined Variables\\Axis 3.Position Feedback"(w284) -> ()  [unwired: 1 in, 1 out]
    n159 = shared-variable "NI-sbRIO9606-018BB5CF\\User-Defined Variables\\Axis 4.Position Feedback"(w283) -> ()  [unwired: 1 in, 1 out]
    n160 = shared-variable "NI-sbRIO9606-018BB5CF\\User-Defined Variables\\Axis 5.Position Feedback"(w282) -> ()  [unwired: 1 in, 1 out]
    n161 = case shown="True" "STEP or CW? (T=STEP)" {
      tunnel: w309 -> [w343 w363]
      tunnel: w308 -> [w342 w353]
      tunnel: w307 -> [w341 w361]
      tunnel: w306 -> [w340 w351]
      tunnel: w305 -> [w339 w359]
      tunnel: w304 -> [w338 w349]
      tunnel: w303 -> [w337 w357]
      tunnel: w302 -> [w336 w347]
      tunnel: w301 -> [w335 w355]
      tunnel: w300 -> [w334 w345]
      tunnel: "Invert direction?" -> [w323 w364]
      tunnel: [w333 w362] -> w298
      tunnel: [w332 w352] -> w289
      tunnel: [w331 w360] -> w297
      tunnel: [w330 w350] -> w296
      tunnel: [w329 w358] -> w295
      tunnel: [w328 w348] -> w294
      tunnel: [w327 w356] -> w293
      tunnel: [w326 w346] -> w292
      tunnel: [w325 w354] -> w291
      tunnel: [w324 w344] -> w290
      frame False {
        n162 = call "Step_Dir_to_CW_CCW.vi"("invert"=w323, "step"=w342, "direction"=w343) -> ("CCW"=w332:bool, "CW"=w333:bool)  [unwired: 7 in]
        n163 = call "Step_Dir_to_CW_CCW.vi"("invert"=w323, "step"=w340, "direction"=w341) -> ("CCW"=w330:bool, "CW"=w331:bool)  [unwired: 7 in]
        n164 = call "Step_Dir_to_CW_CCW.vi"("invert"=w323, "step"=w338, "direction"=w339) -> ("CCW"=w328:bool, "CW"=w329:bool)  [unwired: 7 in]
        n165 = call "Step_Dir_to_CW_CCW.vi"("invert"=w323, "step"=w336, "direction"=w337) -> ("CCW"=w326:bool, "CW"=w327:bool)  [unwired: 7 in]
        n166 = call "Step_Dir_to_CW_CCW.vi"("invert"=w323, "step"=w334, "direction"=w335) -> ("CCW"=w324:bool, "CW"=w325:bool)  [unwired: 7 in]
      }
      frame True {
        n167 = case shown="True" w364 {
          tunnel: w363 -> [w374 w389]
          tunnel: [w374 w388] -> w362
          tunnel: w361 -> [w372 w387]
          tunnel: [w372 w386] -> w360
          tunnel: w359 -> [w370 w385]
          tunnel: [w370 w384] -> w358
          tunnel: w357 -> [w368 w383]
          tunnel: [w368 w382] -> w356
          tunnel: w355 -> [w366 w381]
          tunnel: [w366 w380] -> w354
          tunnel: w353 -> [w373 w379]
          tunnel: [w373 w379] -> w352
          tunnel: w351 -> [w371 w378]
          tunnel: [w371 w378] -> w350
          tunnel: w349 -> [w369 w377]
          tunnel: [w369 w377] -> w348
          tunnel: w347 -> [w367 w376]
          tunnel: [w367 w376] -> w346
          tunnel: w345 -> [w365 w375]
          tunnel: [w365 w375] -> w344
          frame False {
          }
          frame True {
            n168 = Not(x=w389) -> (.not. x?=w388:bool)
            n169 = Not(x=w387) -> (.not. x?=w386:bool)
            n170 = Not(x=w385) -> (.not. x?=w384:bool)
            n171 = Not(x=w383) -> (.not. x?=w382:bool)
            n172 = Not(x=w381) -> (.not. x?=w380:bool)
          }
        }
      }
    }
    n173 = xnode "FPGA I/O Node"("Axis1_CW"=w298, "Axis1_CCW"=w289, "Axis2_CW"=w297, "Axis2_CCW"=w296, "Axis3_CW"=w295, "Axis3_CCW"=w294, "Axis4_CW"=w293, "Axis4_CCW"=w292, "Axis5_CW"=w291, "Axis5_CCW"=w290) -> ()  [unwired: 10 in, 10 out]
  }
  n174 = timed-loop "Synchronization Loop" {
    timing: w5 -> [_]
    timing-out: [_] -> w4
    stop <- FALSE stop-if-true
    n175 = xnode "FPGA I/O Node"() -> ("Scan Clock"=w396:bool)  [unwired: 1 in, 1 out]
    n176 = global read "Global FPGA.vi" "Sync Enable"() -> (w395:bool)
    n177 = Select(t="Sync Value", s="Sync Enable override?", f=w395) -> (s? t:f=w392:bool)
    n178 = call-poly <vilib>:"nism.scan.generateSyncScan.vi"("Scan Enable?"=w392, "Scan Clock"=w396) -> ("Timer Control"=w397:T10)  [unwired: 3 in]
    n179 = global write "Global FPGA.vi" "Timer Control"(w397) -> ()
  }
  n180 = timed-loop "Reset Monitoring Loop" {
    timing: w3 -> [_]
    timing-out: [_] -> w2
    stop <- FALSE stop-if-true
    n181 = global read "Global FPGA.vi" "Reset Pending"() -> (w403:bool[])
    n182 = xnode "FPGA I/O Node"() -> ("Scan Clock"=w402:bool)  [unwired: 1 in, 1 out]
    n183 = feedback-in #2(w402) -> ()
    n184 = feedback #2() -> (w401:bool)  [unwired: 1 in]
    n185 = Greater?(x=w402, y=w401) -> (0:w407:bool)
    n186 = feedback #3() -> (w406:bool[])  [unwired: 1 in]
    n187 = Select(t=w403, s=w407, f=w406) -> (s? t:f=w404:bool[])
    n188 = feedback-in #3(w404) -> ()
    n189 = global write "Global FPGA.vi" "Reset"(w404) -> ()
  }
  n190 = node-c288(w2) -> ()
  n191 = node-c288(w4) -> ()
  n192 = node-c288(w6) -> ()
